vi "Read.vi"(8 "error in (no error)":errorcluster, 11 "Double Float.lvclass_340760 in":refnum<class "Abs_Double Float 1D.lvclass">) -> (0 "error out":errorcluster, 2 "Value":T1, 3 "Double Float.lvclass_340760 out":refnum<class "Abs_Double Float 1D.lvclass">)   [LabVIEW 2021, in "Abs_Double Float 1D.lvclass"]
uses:
  Abs_Double Float 1D.lvclass
  Support/Type.ctl
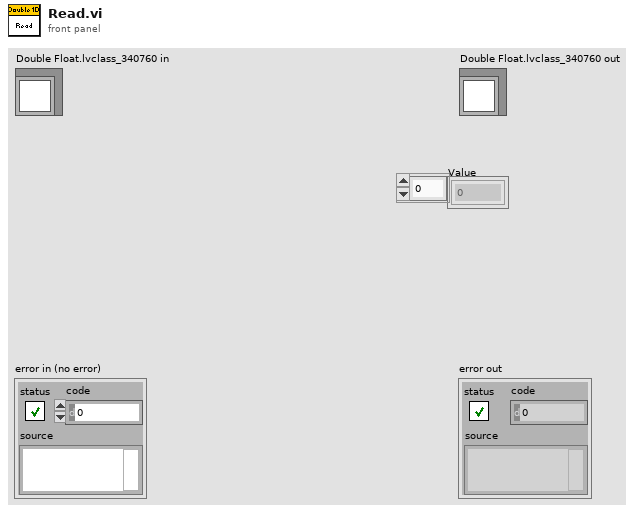
[diagram p1: front panel]
types:
  T1 = typedef "Abs_Double Float 1D.lvclass/Type.ctl" = dbl[]
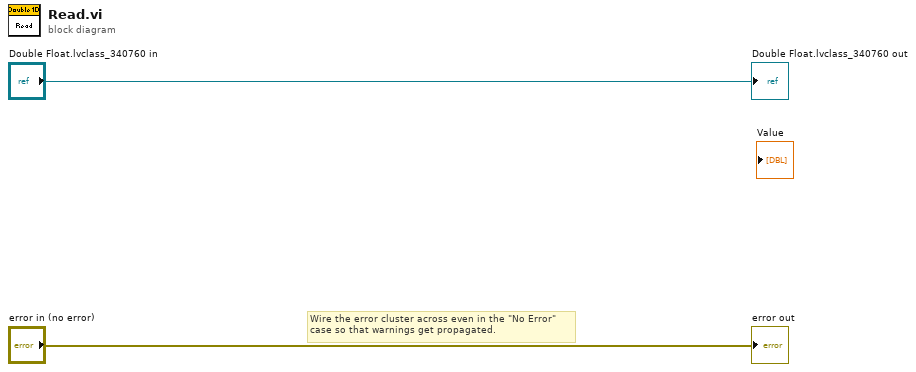
[diagram p0: block diagram]
diagram:
  # "Wire the error cluster across even in the \"No Error\"\ncase so that warnings get propagated."
  "error out" <- "error in (no error)"
  "Double Float.lvclass_340760 out" <- "Double Float.lvclass_340760 in"
